vi "aFGV - Read Write Config File.vi"(6 "State":enum16{"Read", "Write", "Delete"}(ring), 7 "Section":T1, 8 "Error In":errorcluster, 9 "Path File":cluster{"Path Out":path, "Filename":string}, 10 "Key Names In":string[](array[string]), 11 "Data in":string[](array[string])) -> (0 "Error Out":errorcluster, 2 "Key Names Out":string[](array[string]), 3 "Data out":string[](array[string]))   [LabVIEW 2020]
uses:
  Control/Config File Section List.ctl
  <vilib>/Utility/config.llb/Read Key (String).vi
  <vilib>/Utility/config.llb/Write Key (String).vi
  <vilib>/Utility/config.llb/NI_LVConfig.lvlib
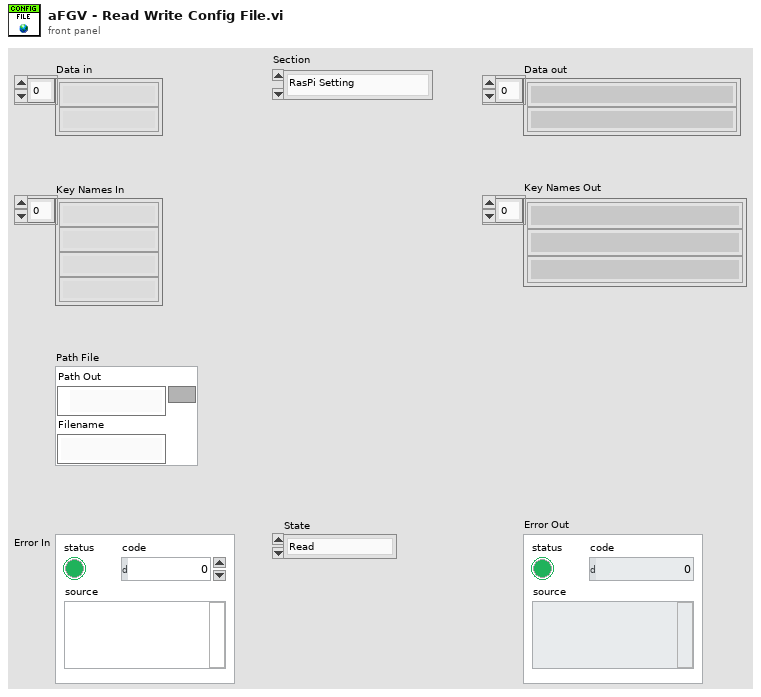
[diagram p1: front panel]
types:
  T1 = typedef "Config File Section List.ctl" = enum16{"RasPi Setting", "MQTT Server Setting", "MQTT Client Setting", "WiFi Setting", "MQTT Topics"}
  T2 = typedef "NI_LVConfig.lvlib/Config Data RefNum.ctl" = refnum<k1>
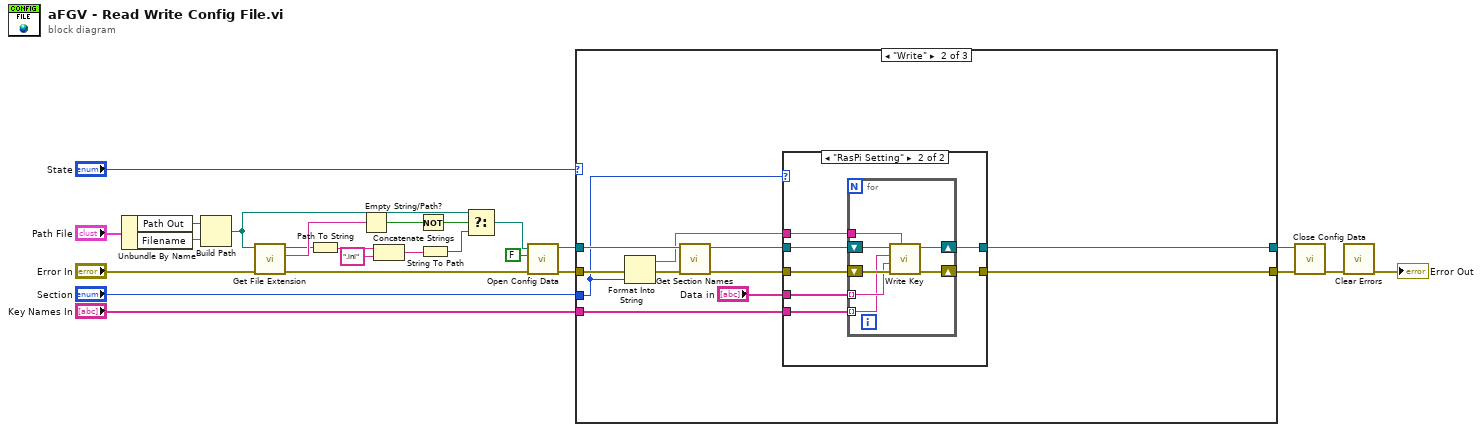
[diagram p0: block diagram]
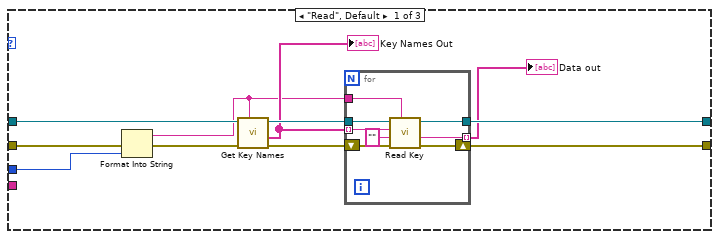
[diagram p2: hidden frame]
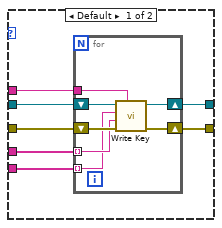
[diagram p3: hidden frame]
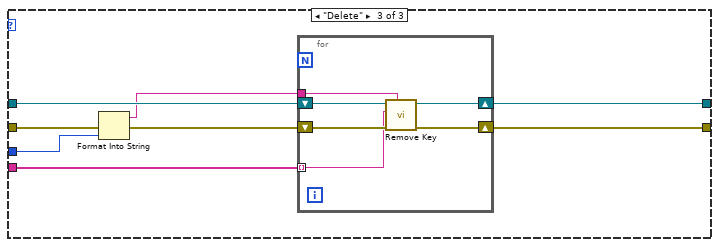
[diagram p4: hidden frame]
diagram:
  n1 = Unbundle By Name("Path File") -> ("Path Out"=w14:path, "Filename"=w13:string)
  n2 = Build Path(base path=w14, name or relative path=w13) -> (appended path=w3:path)
  n3 = call <vilib>:"Get File Extension.vi"("error in (no error)"="Error In", "file"=w3) -> ("error out"=w4:errorcluster, "lowercase file extension"=w12:string, "dup file"=w2:path)  [unwired: 5 in, 2 out]
  n4 = Path To String(path=w2) -> (string=w11:string)
  n5 = Empty String/Path?(string/path=w12) -> (empty?=w8:bool)
  n6 = Concatenate Strings(w11, ".ini" ("string")) -> (w9:string)
  n7 = Not(x=w8) -> (.not. x?=w1:bool)
  n8 = String To Path(string=w9) -> (path=w7:path)
  n9 = Select(t=w3, s=w1, f=w7) -> (s? t:f=w6:path)
  n10 = call <vilib>:"Open Config Data.vi"("error in (no error)"=w4, "create file if necessary (T)"=FALSE, "configuration file path"=w6) -> ("error out"=w25:errorcluster, "refnum"=w21:T2)  [unwired: 6 in, 1 out]
  n11 = case shown="\"Write\"" "State" {
    tunnel: w25 -> [w33 w55 w91]
    tunnel: w21 -> [w32 w51 w88]
    tunnel: [w36 w54 w90] -> w24
    tunnel: [w31 w50 w87] -> w20
    tunnel: "Section" -> [w27 w47 w86]
    tunnel: "Key Names In" -> [_ w45 w84]
    frame "Read", Default {
      n12 = Format Into String(error in=w33, w27) -> (resulting string=w26:string, error out=w34:errorcluster)  [unwired: 2 in]
      n13 = call <vilib>:"Get Key Names.vi"("section"=w26, "error in (no error)"=w34, "refnum"=w32) -> ("error out"=w35:errorcluster, "key names"=w29:string[], "refnum out"=w30:T2)  [unwired: 5 in, 1 out]
      "Key Names Out" <- w29
      n14 = for {
        tunnel: w30 -> [w42]
        shift-right: [w44] -> w36
        shift-left: w35 -> [w43]
        tunnel: w29 -> [w41] mode=indexing
        tunnel: w26 -> [w39]
        tunnel: [w38] -> w31
        tunnel: [w37] -> w28 mode=indexing
        n15 = call-poly <vilib>:"Read Key.vi"("section"=w39, "error in (no error)"=w43, "default value"="", "key"=w41, "refnum"=w42) -> ("error out"=w44:errorcluster, "value"=w37:string, "refnum out"=w38:T2)  [unwired: 3 in, 1 out]
      }
      "Data out" <- w28
    }
    frame "Write" {
      n16 = Format Into String(error in=w55, w47) -> (resulting string=w46:string, error out=w52:errorcluster)  [unwired: 2 in]
      n17 = call <vilib>:"Get Section Names.vi"("error in (no error)"=w52, "refnum"=w51) -> ("error out"=w53:errorcluster, "refnum out"=w49:T2)  [unwired: 7 in, 1 out]
      n18 = case shown="\"RasPi Setting\"" w47 {
        tunnel: w53 -> [w62 w76]
        tunnel: [w61 w75] -> w54
        tunnel: w46 -> [w60 w74]
        tunnel: w49 -> [w59 w73]
        tunnel: [w58 w72] -> w50
        tunnel: "Data in" -> [w57 w71]
        tunnel: w45 -> [w56 w70]
        frame Default {
          n19 = for {
            tunnel: w60 -> [w67]
            tunnel: w57 -> [w64] mode=indexing
            shift-right: [w68] -> w61
            shift-left: w62 -> [w69]
            shift-right: [w65] -> w58
            shift-left: w59 -> [w66]
            tunnel: w56 -> [w63] mode=indexing
            n20 = call-poly <vilib>:"Write Key.vi"("section"=w67, "error in (no error)"=w69, "value"=w64, "key"=w63, "refnum"=w66) -> ("error out"=w68:errorcluster, "refnum out"=w65:T2)  [unwired: 4 in, 1 out]
          }
        }
        frame "RasPi Setting" {
          n21 = for {
            tunnel: w74 -> [w81]
            tunnel: w71 -> [w78] mode=indexing
            shift-right: [w82] -> w75
            shift-left: w76 -> [w83]
            shift-right: [w79] -> w72
            shift-left: w73 -> [w80]
            tunnel: w70 -> [w77] mode=indexing
            n22 = call-poly <vilib>:"Write Key.vi"("section"=w81, "error in (no error)"=w83, "value"=w78, "key"=w77, "refnum"=w80) -> ("error out"=w82:errorcluster, "refnum out"=w79:T2)  [unwired: 4 in, 1 out]
          }
        }
      }
    }
    frame "Delete" {
      n23 = Format Into String(error in=w91, w86) -> (resulting string=w85:string, error out=w89:errorcluster)  [unwired: 2 in]
      n24 = for {
        tunnel: w85 -> [w93]
        tunnel: w84 -> [w92] mode=indexing
        shift-right: [w97] -> w90
        shift-left: w89 -> [w96]
        shift-right: [w94] -> w87
        shift-left: w88 -> [w95]
        n25 = call <vilib>:"Remove Key.vi"("section"=w93, "error in (no error)"=w96, "key"=w92, "refnum"=w95) -> ("error out"=w97:errorcluster, "refnum out"=w94:T2)  [unwired: 5 in, 1 out]
      }
    }
  }
  n26 = call <vilib>:"Close Config Data.vi"("error in (no error)"=w24, "refnum"=w20) -> ("error out"=w23:errorcluster)  [unwired: 8 in, 1 out]
  n27 = call <vilib>:"Clear Errors.vi"("error in (no error)"=w23) -> ("error out"=→"Error Out":errorcluster)  [unwired: 5 in, 1 out]
